vi "DDS_Clock.vi"() -> ()   [LabVIEW 2016] (continued)
 [Hz] CH0"=316600000.0}, {"total time[ms]"=45.84999999999953, "f1 [Hz] CH0"=316600000.0}, {"total time[ms]"=45.89999999999953, "f1 [Hz] CH0"=316400000.0}, {"total time[ms]"=45.89999999999953, "f1 [Hz] CH0"=316400000.0}, {"total time[ms]"=45.94999999999953, "f1 [Hz] CH0"=316200000.0}, {"total time[ms]"=45.94999999999953, "f1 [Hz] CH0"=316200000.0}, {"total time[ms]"=45.999999999999524, "f1 [Hz] CH0"=316000000.0}, {"total time[ms]"=45.999999999999524, "f1 [Hz] CH0"=316000000.0}, {"total time[ms]"=46.04999999999952, "f1 [Hz] CH0"=315800000.0}, {"total time[ms]"=46.04999999999952, "f1 [Hz] CH0"=315800000.0}, {"total time[ms]"=46.09999999999952, "f1 [Hz] CH0"=315600000.0}, {"total time[ms]"=46.09999999999952, "f1 [Hz] CH0"=315600000.0}, {"total time[ms]"=46.149999999999515, "f1 [Hz] CH0"=315399999.99999994}, {"total time[ms]"=46.149999999999515, "f1 [Hz] CH0"=315399999.99999994}, {"total time[ms]"=46.19999999999951, "f1 [Hz] CH0"=315200000.0}, {"total time[ms]"=46.19999999999951, "f1 [Hz] CH0"=315200000.0}, {"total time[ms]"=46.24999999999951, "f1 [Hz] CH0"=315000000.0}, {"total time[ms]"=46.24999999999951, "f1 [Hz] CH0"=315000000.0}, {"total time[ms]"=46.29999999999951, "f1 [Hz] CH0"=314799999.99999994}, {"total time[ms]"=46.29999999999951, "f1 [Hz] CH0"=314799999.99999994}, {"total time[ms]"=46.349999999999504, "f1 [Hz] CH0"=314600000.0}, {"total time[ms]"=46.349999999999504, "f1 [Hz] CH0"=314600000.0}, {"total time[ms]"=46.3999999999995, "f1 [Hz] CH0"=314400000.0}, {"total time[ms]"=46.3999999999995, "f1 [Hz] CH0"=314400000.0}, {"total time[ms]"=46.4499999999995, "f1 [Hz] CH0"=314200000.0}, {"total time[ms]"=46.4499999999995, "f1 [Hz] CH0"=314200000.0}, {"total time[ms]"=46.499999999999496, "f1 [Hz] CH0"=314000000.0}, {"total time[ms]"=46.499999999999496, "f1 [Hz] CH0"=314000000.0}, {"total time[ms]"=46.54999999999949, "f1 [Hz] CH0"=313800000.0}, {"total time[ms]"=46.54999999999949, "f1 [Hz] CH0"=313800000.0}, {"total time[ms]"=46.59999999999949, "f1 [Hz] CH0"=313600000.0}, {"total time[ms]"=46.59999999999949, "f1 [Hz] CH0"=313600000.0}, {"total time[ms]"=46.64999999999949, "f1 [Hz] CH0"=313399999.99999994}, {"total time[ms]"=46.64999999999949, "f1 [Hz] CH0"=313399999.99999994}, {"total time[ms]"=46.699999999999484, "f1 [Hz] CH0"=313199999.99999994}, {"total time[ms]"=46.699999999999484, "f1 [Hz] CH0"=313199999.99999994}, {"total time[ms]"=46.74999999999948, "f1 [Hz] CH0"=313000000.0}, {"total time[ms]"=46.74999999999948, "f1 [Hz] CH0"=313000000.0}, {"total time[ms]"=46.79999999999948, "f1 [Hz] CH0"=312800000.0}, {"total time[ms]"=46.79999999999948, "f1 [Hz] CH0"=312800000.0}, {"total time[ms]"=46.849999999999476, "f1 [Hz] CH0"=312600000.0}, {"total time[ms]"=46.849999999999476, "f1 [Hz] CH0"=312600000.0}, {"total time[ms]"=46.89999999999947, "f1 [Hz] CH0"=312400000.0}, {"total time[ms]"=46.89999999999947, "f1 [Hz] CH0"=312400000.0}, {"total time[ms]"=46.94999999999947, "f1 [Hz] CH0"=312200000.0}, {"total time[ms]"=46.94999999999947, "f1 [Hz] CH0"=312200000.0}, {"total time[ms]"=46.99999999999947, "f1 [Hz] CH0"=312000000.0}, {"total time[ms]"=46.99999999999947, "f1 [Hz] CH0"=312000000.0}, {"total time[ms]"=47.049999999999464, "f1 [Hz] CH0"=311799999.99999994}, {"total time[ms]"=47.049999999999464, "f1 [Hz] CH0"=311799999.99999994}, {"total time[ms]"=47.09999999999946, "f1 [Hz] CH0"=311600000.0}, {"total time[ms]"=47.09999999999946, "f1 [Hz] CH0"=311600000.0}, {"total time[ms]"=47.14999999999946, "f1 [Hz] CH0"=311400000.0}, {"total time[ms]"=47.14999999999946, "f1 [Hz] CH0"=311400000.0}, {"total time[ms]"=47.199999999999456, "f1 [Hz] CH0"=311200000.0}, {"total time[ms]"=47.199999999999456, "f1 [Hz] CH0"=311200000.0}, {"total time[ms]"=47.24999999999945, "f1 [Hz] CH0"=311000000.0}, {"total time[ms]"=47.24999999999945, "f1 [Hz] CH0"=311000000.0}, {"total time[ms]"=47.29999999999945, "f1 [Hz] CH0"=310800000.0}, {"total time[ms]"=47.29999999999945, "f1 [Hz] CH0"=310800000.0}, {"total time[ms]"=47.34999999999945, "f1 [Hz] CH0"=310600000.0}, {"total time[ms]"=47.34999999999945, "f1 [Hz] CH0"=310600000.0}, {"total time[ms]"=47.399999999999444, "f1 [Hz] CH0"=310399999.99999994}, {"total time[ms]"=47.399999999999444, "f1 [Hz] CH0"=310399999.99999994}, {"total time[ms]"=47.44999999999944, "f1 [Hz] CH0"=310200000.0}, {"total time[ms]"=47.44999999999944, "f1 [Hz] CH0"=310200000.0}, {"total time[ms]"=47.49999999999944, "f1 [Hz] CH0"=310000000.0}, {"total time[ms]"=47.49999999999944, "f1 [Hz] CH0"=310000000.0}, {"total time[ms]"=47.549999999999436, "f1 [Hz] CH0"=309799999.99999994}, {"total time[ms]"=47.549999999999436, "f1 [Hz] CH0"=309799999.99999994}, {"total time[ms]"=47.59999999999943, "f1 [Hz] CH0"=309600000.0}, {"total time[ms]"=47.59999999999943, "f1 [Hz] CH0"=309600000.0}, {"total time[ms]"=47.64999999999943, "f1 [Hz] CH0"=309400000.0}, {"total time[ms]"=47.64999999999943, "f1 [Hz] CH0"=309400000.0}, {"total time[ms]"=47.69999999999943, "f1 [Hz] CH0"=309200000.0}, {"total time[ms]"=47.69999999999943, "f1 [Hz] CH0"=309200000.0}, {"total time[ms]"=47.749999999999424, "f1 [Hz] CH0"=309000000.0}, {"total time[ms]"=47.749999999999424, "f1 [Hz] CH0"=309000000.0}, {"total time[ms]"=47.79999999999942, "f1 [Hz] CH0"=308800000.0}, {"total time[ms]"=47.79999999999942, "f1 [Hz] CH0"=308800000.0}, {"total time[ms]"=47.84999999999942, "f1 [Hz] CH0"=308600000.0}, {"total time[ms]"=47.84999999999942, "f1 [Hz] CH0"=308600000.0}, {"total time[ms]"=47.899999999999416, "f1 [Hz] CH0"=308399999.99999994}, {"total time[ms]"=47.899999999999416, "f1 [Hz] CH0"=308399999.99999994}, {"total time[ms]"=47.94999999999941, "f1 [Hz] CH0"=308199999.99999994}, {"total time[ms]"=47.94999999999941, "f1 [Hz] CH0"=308199999.99999994}, {"total time[ms]"=47.99999999999941, "f1 [Hz] CH0"=308000000.0}, {"total time[ms]"=47.99999999999941, "f1 [Hz] CH0"=308000000.0}, {"total time[ms]"=48.04999999999941, "f1 [Hz] CH0"=307800000.0}, {"total time[ms]"=48.04999999999941, "f1 [Hz] CH0"=307800000.0}, {"total time[ms]"=48.099999999999405, "f1 [Hz] CH0"=307600000.0}, {"total time[ms]"=48.099999999999405, "f1 [Hz] CH0"=307600000.0}, {"total time[ms]"=48.1499999999994, "f1 [Hz] CH0"=307399999.99999994}, {"total time[ms]"=48.1499999999994, "f1 [Hz] CH0"=307399999.99999994}, {"total time[ms]"=48.1999999999994, "f1 [Hz] CH0"=307200000.0}, {"total time[ms]"=48.1999999999994, "f1 [Hz] CH0"=307200000.0}, {"total time[ms]"=48.249999999999396, "f1 [Hz] CH0"=307000000.0}, {"total time[ms]"=48.249999999999396, "f1 [Hz] CH0"=307000000.0}, {"total time[ms]"=48.29999999999939, "f1 [Hz] CH0"=306799999.99999994}, {"total time[ms]"=48.29999999999939, "f1 [Hz] CH0"=306799999.99999994}, {"total time[ms]"=48.34999999999939, "f1 [Hz] CH0"=306599999.99999994}, {"total time[ms]"=48.34999999999939, "f1 [Hz] CH0"=306599999.99999994}, {"total time[ms]"=48.39999999999939, "f1 [Hz] CH0"=306400000.0}, {"total time[ms]"=48.39999999999939, "f1 [Hz] CH0"=306400000.0}, {"total time[ms]"=48.449999999999385, "f1 [Hz] CH0"=306200000.0}, {"total time[ms]"=48.449999999999385, "f1 [Hz] CH0"=306200000.0}, {"total time[ms]"=48.49999999999938, "f1 [Hz] CH0"=306000000.0}, {"total time[ms]"=48.49999999999938, "f1 [Hz] CH0"=306000000.0}, {"total time[ms]"=48.54999999999938, "f1 [Hz] CH0"=305800000.0}, {"total time[ms]"=48.54999999999938, "f1 [Hz] CH0"=305800000.0}, {"total time[ms]"=48.599999999999376, "f1 [Hz] CH0"=305600000.0}, {"total time[ms]"=48.599999999999376, "f1 [Hz] CH0"=305600000.0}, {"total time[ms]"=48.64999999999937, "f1 [Hz] CH0"=305399999.99999994}, {"total time[ms]"=48.64999999999937, "f1 [Hz] CH0"=305399999.99999994}, {"total time[ms]"=48.69999999999937, "f1 [Hz] CH0"=305199999.99999994}, {"total time[ms]"=48.69999999999937, "f1 [Hz] CH0"=305199999.99999994}, {"total time[ms]"=48.74999999999937, "f1 [Hz] CH0"=305000000.0}, {"total time[ms]"=48.74999999999937, "f1 [Hz] CH0"=305000000.0}, {"total time[ms]"=48.799999999999365, "f1 [Hz] CH0"=304799999.99999994}, {"total time[ms]"=48.799999999999365, "f1 [Hz] CH0"=304799999.99999994}, {"total time[ms]"=48.84999999999936, "f1 [Hz] CH0"=304600000.0}, {"total time[ms]"=48.84999999999936, "f1 [Hz] CH0"=304600000.0}, {"total time[ms]"=48.89999999999936, "f1 [Hz] CH0"=304400000.0}, {"total time[ms]"=48.89999999999936, "f1 [Hz] CH0"=304400000.0}, {"total time[ms]"=48.949999999999356, "f1 [Hz] CH0"=304200000.0}, {"total time[ms]"=48.949999999999356, "f1 [Hz] CH0"=304200000.0}, {"total time[ms]"=48.99999999999935, "f1 [Hz] CH0"=304000000.0}, {"total time[ms]"=48.99999999999935, "f1 [Hz] CH0"=304000000.0}, {"total time[ms]"=49.04999999999935, "f1 [Hz] CH0"=303799999.99999994}, {"total time[ms]"=49.04999999999935, "f1 [Hz] CH0"=303799999.99999994}, {"total time[ms]"=49.09999999999935, "f1 [Hz] CH0"=303600000.0}, {"total time[ms]"=49.09999999999935, "f1 [Hz] CH0"=303600000.0}, {"total time[ms]"=49.149999999999345, "f1 [Hz] CH0"=303399999.99999994}, {"total time[ms]"=49.149999999999345, "f1 [Hz] CH0"=303399999.99999994}, {"total time[ms]"=49.19999999999934, "f1 [Hz] CH0"=303199999.99999994}, {"total time[ms]"=49.19999999999934, "f1 [Hz] CH0"=303199999.99999994}, {"total time[ms]"=49.24999999999934, "f1 [Hz] CH0"=303000000.0}, {"total time[ms]"=49.24999999999934, "f1 [Hz] CH0"=303000000.0}, {"total time[ms]"=49.299999999999336, "f1 [Hz] CH0"=302800000.0}, {"total time[ms]"=49.299999999999336, "f1 [Hz] CH0"=302800000.0}, {"total time[ms]"=49.34999999999933, "f1 [Hz] CH0"=302600000.0}, {"total time[ms]"=49.34999999999933, "f1 [Hz] CH0"=302600000.0}, {"total time[ms]"=49.39999999999933, "f1 [Hz] CH0"=302399999.99999994}, {"total time[ms]"=49.39999999999933, "f1 [Hz] CH0"=302399999.99999994}, {"total time[ms]"=49.44999999999933, "f1 [Hz] CH0"=302200000.0}, {"total time[ms]"=49.44999999999933, "f1 [Hz] CH0"=302200000.0}, {"total time[ms]"=49.499999999999325, "f1 [Hz] CH0"=302000000.0}, {"total time[ms]"=49.499999999999325, "f1 [Hz] CH0"=302000000.0}, {"total time[ms]"=49.54999999999932, "f1 [Hz] CH0"=301799999.99999994}, {"total time[ms]"=49.54999999999932, "f1 [Hz] CH0"=301799999.99999994}, {"total time[ms]"=49.59999999999932, "f1 [Hz] CH0"=301599999.99999994}, {"total time[ms]"=49.59999999999932, "f1 [Hz] CH0"=301599999.99999994}, {"total time[ms]"=49.64999999999932, "f1 [Hz] CH0"=301400000.0}, {"total time[ms]"=49.64999999999932, "f1 [Hz] CH0"=301400000.0}, {"total time[ms]"=49.699999999999314, "f1 [Hz] CH0"=301200000.0}, {"total time[ms]"=49.699999999999314, "f1 [Hz] CH0"=301200000.0}, {"total time[ms]"=49.74999999999931, "f1 [Hz] CH0"=301000000.0}, {"total time[ms]"=49.74999999999931, "f1 [Hz] CH0"=301000000.0}, {"total time[ms]"=49.79999999999931, "f1 [Hz] CH0"=300800000.0}, {"total time[ms]"=49.79999999999931, "f1 [Hz] CH0"=300800000.0}, {"total time[ms]"=49.849999999999305, "f1 [Hz] CH0"=300600000.0}, {"total time[ms]"=49.849999999999305, "f1 [Hz] CH0"=300600000.0}, {"total time[ms]"=49.8999999999993, "f1 [Hz] CH0"=300399999.99999994}, {"total time[ms]"=49.8999999999993, "f1 [Hz] CH0"=300399999.99999994}, {"total time[ms]"=49.9499999999993, "f1 [Hz] CH0"=300199999.99999994}, {"total time[ms]"=49.9499999999993, "f1 [Hz] CH0"=300199999.99999994}, {"total time[ms]"=49.9999999999993, "f1 [Hz] CH0"=300000000.0}, {"total time[ms]"=49.9999999999993, "f1 [Hz] CH0"=300000000.0}, {"total time[ms]"=50.049999999999294, "f1 [Hz] CH0"=300200000.00000006}, {"total time[ms]"=50.049999999999294, "f1 [Hz] CH0"=300200000.00000006}, {"total time[ms]"=50.09999999999929, "f1 [Hz] CH0"=300400000.0}, {"total time[ms]"=50.09999999999929, "f1 [Hz] CH0"=300400000.0}, {"total time[ms]"=50.14999999999929, "f1 [Hz] CH0"=300600000.0}, {"total time[ms]"=50.14999999999929, "f1 [Hz] CH0"=300600000.0}, {"total time[ms]"=50.199999999999285, "f1 [Hz] CH0"=300800000.0}, {"total time[ms]"=50.199999999999285, "f1 [Hz] CH0"=300800000.0}, {"total time[ms]"=50.24999999999928, "f1 [Hz] CH0"=301000000.0}, {"total time[ms]"=50.24999999999928, "f1 [Hz] CH0"=301000000.0}, {"total time[ms]"=50.29999999999928, "f1 [Hz] CH0"=301200000.00000006}, {"total time[ms]"=50.29999999999928, "f1 [Hz] CH0"=301200000.00000006}, {"total time[ms]"=50.34999999999928, "f1 [Hz] CH0"=301400000.0}, {"total time[ms]"=50.34999999999928, "f1 [Hz] CH0"=301400000.0}, {"total time[ms]"=50.399999999999274, "f1 [Hz] CH0"=301600000.00000006}, {"total time[ms]"=50.399999999999274, "f1 [Hz] CH0"=301600000.00000006}, {"total time[ms]"=50.44999999999927, "f1 [Hz] CH0"=301800000.00000006}, {"total time[ms]"=50.44999999999927, "f1 [Hz] CH0"=301800000.00000006}, {"total time[ms]"=50.49999999999927, "f1 [Hz] CH0"=302000000.0}, {"total time[ms]"=50.49999999999927, "f1 [Hz] CH0"=302000000.0}, {"total time[ms]"=50.549999999999265, "f1 [Hz] CH0"=302200000.0}, {"total time[ms]"=50.549999999999265, "f1 [Hz] CH0"=302200000.0}, {"total time[ms]"=50.59999999999926, "f1 [Hz] CH0"=302400000.0}, {"total time[ms]"=50.59999999999926, "f1 [Hz] CH0"=302400000.0}, {"total time[ms]"=50.64999999999926, "f1 [Hz] CH0"=302600000.00000006}, {"total time[ms]"=50.64999999999926, "f1 [Hz] CH0"=302600000.00000006}, {"total time[ms]"=50.69999999999926, "f1 [Hz] CH0"=302800000.0}, {"total time[ms]"=50.69999999999926, "f1 [Hz] CH0"=302800000.0}, {"total time[ms]"=50.749999999999254, "f1 [Hz] CH0"=303000000.0}, {"total time[ms]"=50.749999999999254, "f1 [Hz] CH0"=303000000.0}, {"total time[ms]"=50.79999999999925, "f1 [Hz] CH0"=303200000.00000006}, {"total time[ms]"=50.79999999999925, "f1 [Hz] CH0"=303200000.00000006}, {"total time[ms]"=50.84999999999925, "f1 [Hz] CH0"=303400000.00000006}, {"total time[ms]"=50.84999999999925, "f1 [Hz] CH0"=303400000.00000006}, {"total time[ms]"=50.899999999999245, "f1 [Hz] CH0"=303600000.0}, {"total time[ms]"=50.899999999999245, "f1 [Hz] CH0"=303600000.0}, {"total time[ms]"=50.94999999999924, "f1 [Hz] CH0"=303800000.0}, {"total time[ms]"=50.94999999999924, "f1 [Hz] CH0"=303800000.0}, {"total time[ms]"=50.99999999999924, "f1 [Hz] CH0"=304000000.0}, {"total time[ms]"=50.99999999999924, "f1 [Hz] CH0"=304000000.0}, {"total time[ms]"=51.04999999999924, "f1 [Hz] CH0"=304200000.0}, {"total time[ms]"=51.04999999999924, "f1 [Hz] CH0"=304200000.0}, {"total time[ms]"=51.099999999999234, "f1 [Hz] CH0"=304400000.0}, {"total time[ms]"=51.099999999999234, "f1 [Hz] CH0"=304400000.0}, {"total time[ms]"=51.14999999999923, "f1 [Hz] CH0"=304600000.00000006}, {"total time[ms]"=51.14999999999923, "f1 [Hz] CH0"=304600000.00000006}, {"total time[ms]"=51.19999999999923, "f1 [Hz] CH0"=304800000.00000006}, {"total time[ms]"=51.19999999999923, "f1 [Hz] CH0"=304800000.00000006}, {"total time[ms]"=51.249999999999226, "f1 [Hz] CH0"=305000000.0}, {"total time[ms]"=51.249999999999226, "f1 [Hz] CH0"=305000000.0}, {"total time[ms]"=51.29999999999922, "f1 [Hz] CH0"=305200000.00000006}, {"total time[ms]"=51.29999999999922, "f1 [Hz] CH0"=305200000.00000006}, {"total time[ms]"=51.34999999999922, "f1 [Hz] CH0"=305400000.0}, {"total time[ms]"=51.34999999999922, "f1 [Hz] CH0"=305400000.0}, {"total time[ms]"=51.39999999999922, "f1 [Hz] CH0"=305600000.0}, {"total time[ms]"=51.39999999999922, "f1 [Hz] CH0"=305600000.0}, {"total time[ms]"=51.449999999999214, "f1 [Hz] CH0"=305800000.0}, {"total time[ms]"=51.449999999999214, "f1 [Hz] CH0"=305800000.0}, {"total time[ms]"=51.49999999999921, "f1 [Hz] CH0"=306000000.0}, {"total time[ms]"=51.49999999999921, "f1 [Hz] CH0"=306000000.0}, {"total time[ms]"=51.54999999999921, "f1 [Hz] CH0"=306200000.00000006}, {"total time[ms]"=51.54999999999921, "f1 [Hz] CH0"=306200000.00000006}, {"total time[ms]"=51.599999999999206, "f1 [Hz] CH0"=306400000.0}, {"total time[ms]"=51.599999999999206, "f1 [Hz] CH0"=306400000.0}, {"total time[ms]"=51.6499999999992, "f1 [Hz] CH0"=306600000.00000006}, {"total time[ms]"=51.6499999999992, "f1 [Hz] CH0"=306600000.00000006}, {"total time[ms]"=51.6999999999992, "f1 [Hz] CH0"=306800000.00000006}, {"total time[ms]"=51.6999999999992, "f1 [Hz] CH0"=306800000.00000006}, {"total time[ms]"=51.7499999999992, "f1 [Hz] CH0"=307000000.0}, {"total time[ms]"=51.7499999999992, "f1 [Hz] CH0"=307000000.0}, {"total time[ms]"=51.799999999999194, "f1 [Hz] CH0"=307200000.0}, {"total time[ms]"=51.799999999999194, "f1 [Hz] CH0"=307200000.0}, {"total time[ms]"=51.84999999999919, "f1 [Hz] CH0"=307400000.0}, {"total time[ms]"=51.84999999999919, "f1 [Hz] CH0"=307400000.0}, {"total time[ms]"=51.89999999999919, "f1 [Hz] CH0"=307600000.00000006}, {"total time[ms]"=51.89999999999919, "f1 [Hz] CH0"=307600000.00000006}, {"total time[ms]"=51.949999999999186, "f1 [Hz] CH0"=307800000.0}, {"total time[ms]"=51.949999999999186, "f1 [Hz] CH0"=307800000.0}, {"total time[ms]"=51.99999999999918, "f1 [Hz] CH0"=308000000.0}, {"total time[ms]"=51.99999999999918, "f1 [Hz] CH0"=308000000.0}, {"total time[ms]"=52.04999999999918, "f1 [Hz] CH0"=308200000.00000006}, {"total time[ms]"=52.04999999999918, "f1 [Hz] CH0"=308200000.00000006}, {"total time[ms]"=52.09999999999918, "f1 [Hz] CH0"=308400000.00000006}, {"total time[ms]"=52.09999999999918, "f1 [Hz] CH0"=308400000.00000006}, {"total time[ms]"=52.149999999999174, "f1 [Hz] CH0"=308600000.0}, {"total time[ms]"=52.149999999999174, "f1 [Hz] CH0"=308600000.0}, {"total time[ms]"=52.19999999999917, "f1 [Hz] CH0"=308800000.0}, {"total time[ms]"=52.19999999999917, "f1 [Hz] CH0"=308800000.0}, {"total time[ms]"=52.24999999999917, "f1 [Hz] CH0"=309000000.0}, {"total time[ms]"=52.24999999999917, "f1 [Hz] CH0"=309000000.0}, {"total time[ms]"=52.299999999999166, "f1 [Hz] CH0"=309200000.0}, {"total time[ms]"=52.299999999999166, "f1 [Hz] CH0"=309200000.0}, {"total time[ms]"=52.34999999999916, "f1 [Hz] CH0"=309400000.0}, {"total time[ms]"=52.34999999999916, "f1 [Hz] CH0"=309400000.0}, {"total time[ms]"=52.39999999999916, "f1 [Hz] CH0"=309600000.00000006}, {"total time[ms]"=52.39999999999916, "f1 [Hz] CH0"=309600000.00000006}, {"total time[ms]"=52.44999999999916, "f1 [Hz] CH0"=309800000.00000006}, {"total time[ms]"=52.44999999999916, "f1 [Hz] CH0"=309800000.00000006}, {"total time[ms]"=52.499999999999154, "f1 [Hz] CH0"=310000000.0}, {"total time[ms]"=52.499999999999154, "f1 [Hz] CH0"=310000000.0}, {"total time[ms]"=52.54999999999915, "f1 [Hz] CH0"=310200000.00000006}, {"total time[ms]"=52.54999999999915, "f1 [Hz] CH0"=310200000.00000006}, {"total time[ms]"=52.59999999999915, "f1 [Hz] CH0"=310400000.0}, {"total time[ms]"=52.59999999999915, "f1 [Hz] CH0"=310400000.0}, {"total time[ms]"=52.649999999999146, "f1 [Hz] CH0"=310600000.0}, {"total time[ms]"=52.649999999999146, "f1 [Hz] CH0"=310600000.0}, {"total time[ms]"=52.69999999999914, "f1 [Hz] CH0"=310800000.0}, {"total time[ms]"=52.69999999999914, "f1 [Hz] CH0"=310800000.0}, {"total time[ms]"=52.74999999999914, "f1 [Hz] CH0"=311000000.0}, {"total time[ms]"=52.74999999999914, "f1 [Hz] CH0"=311000000.0}, {"total time[ms]"=52.79999999999914, "f1 [Hz] CH0"=311200000.00000006}, {"total time[ms]"=52.79999999999914, "f1 [Hz] CH0"=311200000.00000006}, {"total time[ms]"=52.849999999999135, "f1 [Hz] CH0"=311400000.0}, {"total time[ms]"=52.849999999999135, "f1 [Hz] CH0"=311400000.0}, {"total time[ms]"=52.89999999999913, "f1 [Hz] CH0"=311600000.00000006}, {"total time[ms]"=52.89999999999913, "f1 [Hz] CH0"=311600000.00000006}, {"total time[ms]"=52.94999999999913, "f1 [Hz] CH0"=311800000.00000006}, {"total time[ms]"=52.94999999999913, "f1 [Hz] CH0"=311800000.00000006}, {"total time[ms]"=52.999999999999126, "f1 [Hz] CH0"=312000000.0}, {"total time[ms]"=52.999999999999126, "f1 [Hz] CH0"=312000000.0}, {"total time[ms]"=53.04999999999912, "f1 [Hz] CH0"=312200000.0}, {"total time[ms]"=53.04999999999912, "f1 [Hz] CH0"=312200000.0}, {"total time[ms]"=53.09999999999912, "f1 [Hz] CH0"=312400000.0}, {"total time[ms]"=53.09999999999912, "f1 [Hz] CH0"=312400000.0}, {"total time[ms]"=53.14999999999912, "f1 [Hz] CH0"=312600000.00000006}, {"total time[ms]"=53.14999999999912, "f1 [Hz] CH0"=312600000.00000006}, {"total time[ms]"=53.199999999999115, "f1 [Hz] CH0"=312800000.0}, {"total time[ms]"=53.199999999999115, "f1 [Hz] CH0"=312800000.0}, {"total time[ms]"=53.24999999999911, "f1 [Hz] CH0"=313000000.0}, {"total time[ms]"=53.24999999999911, 
